vi "ReadMerecuryIPS_Ethernet.vi"() -> ()   [LabVIEW 2015]
panel:
  out "Reading of temperature that I still have to figure out which":string
  out "Reading of the He level from the lavel controller board (DB5.L1)":string
  in  "error in (no error)":errorcluster
  out "error out":errorcluster
  out "Reading of magnetic field":string
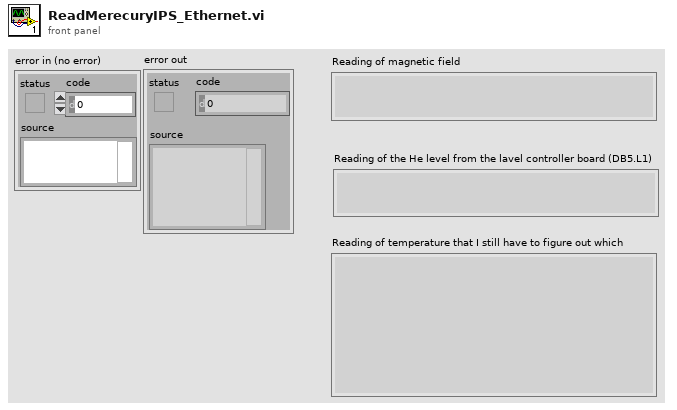
[diagram p1: front panel]
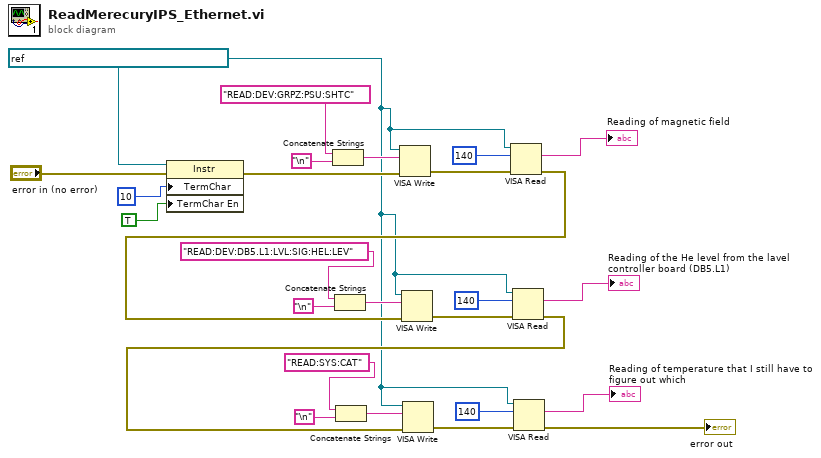
[diagram p0: block diagram]
diagram:
  w1 = refnum<visa-resource-name> "TCPIP0::192.168.128.3::7020::SOCKET" ("VISA resource name")
  n1 = property class="Instr"(reference=w1, error in="error in (no error)", "TermChar"=10, "TermChar En"=TRUE) -> (error out=w11:errorcluster)  [unwired: 1 out]
  n2 = Concatenate Strings("READ:DEV:GRPZ:PSU:SHTC" ("string"), "\n") -> (w23:string)
  n3 = Concatenate Strings("READ:DEV:DB5.L1:LVL:SIG:HEL:LEV" ("string"), "\n") -> (w16:string)
  n4 = Concatenate Strings("READ:SYS:CAT" ("string"), "\n") -> (w6:string)
  n5 = VISA Write(VISA resource name=w1, write buffer=w23, error in (no error)=w11) -> (error out=w26:errorcluster)  [unwired: 2 out]
  n6 = VISA Read(VISA resource name=w1, byte count=140, error in (no error)=w26) -> (read buffer=→"Reading of magnetic field":string, error out=w13:errorcluster)  [unwired: 2 out]
  n7 = VISA Write(VISA resource name=w1, write buffer=w16, error in (no error)=w13) -> (error out=w19:errorcluster)  [unwired: 2 out]
  n8 = VISA Read(VISA resource name=w1, byte count=140, error in (no error)=w19) -> (read buffer=→"Reading of the He level from the lavel controller board (DB5.L1)":string, error out=w2:errorcluster)  [unwired: 2 out]
  n9 = VISA Write(VISA resource name=w1, write buffer=w6, error in (no error)=w2) -> (error out=w9:errorcluster)  [unwired: 2 out]
  n10 = VISA Read(VISA resource name=w1, byte count=140, error in (no error)=w9) -> (read buffer=→"Reading of temperature that I still have to figure out which":string, error out=→"error out":errorcluster)  [unwired: 2 out]
